vi "Contour Line_Find Candidate Edges.vi"(11 "edge":T2) -> (3 "Candidate Edges":T1(array[cluster]))   [LabVIEW 2020, in "NI_AAL_Geometry.lvlib"]
uses:
  <vilib>/Analysis/NI_AAL_Geometry.lvlib
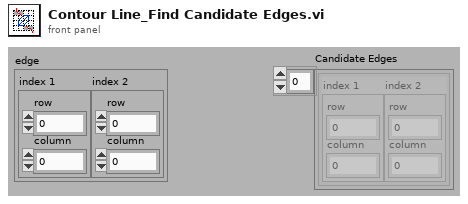
[diagram p1: front panel]
types:
  T1 = cluster{"index 1":cluster{"row":i32, "column":i32}, "index 2":cluster{"row":i32, "column":i32}}[]
  T2 = cluster{"index 1":cluster{"row":i32, "column":i32}, "index 2":cluster{"row":i32, "column":i32}}
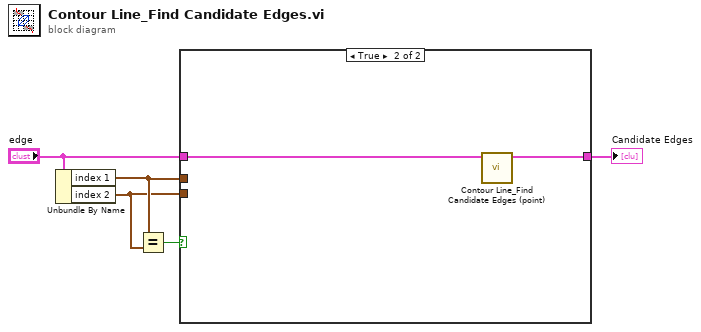
[diagram p0: block diagram]
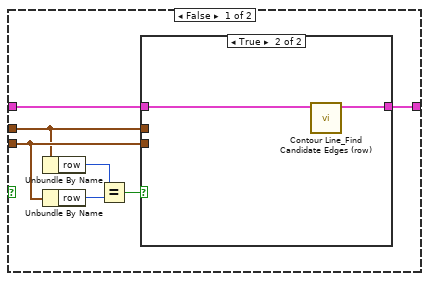
[diagram p2: hidden frame]
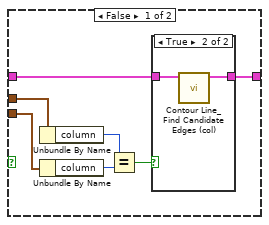
[diagram p3: hidden frame]
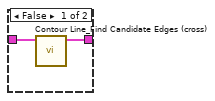
[diagram p4: hidden frame]
diagram:
  n1 = Unbundle By Name("edge") -> ("index 1"=w4:cluster{"row":i32, "column":i32}, "index 2"=w3:cluster{"row":i32, "column":i32})
  n2 = Equal?(x=w4, y=w3) -> (x = y?=w2:bool)
  n3 = case shown="True" w2 {
    tunnel: "edge" -> [w7 w27]
    tunnel: w4 -> [w8 _]
    tunnel: w3 -> [w9 _]
    tunnel: [w6 w26] -> w1
    frame False {
      n4 = Unbundle By Name(w8) -> ("row"=w11:i32)
      n5 = Unbundle By Name(w9) -> ("row"=w12:i32)
      n6 = Equal?(x=w11, y=w12) -> (x = y?=w10:bool)
      n7 = case shown="True" w10 {
        tunnel: w9 -> [w16 _]
        tunnel: w8 -> [w17 _]
        tunnel: w7 -> [w14 w25]
        tunnel: [w13 w24] -> w6
        frame False {
          n8 = Unbundle By Name(w17) -> ("column"=w19:i32)
          n9 = Unbundle By Name(w16) -> ("column"=w18:i32)
          n10 = Equal?(x=w19, y=w18) -> (x = y?=w15:bool)
          n11 = case shown="True" w15 {
            tunnel: w14 -> [w21 w23]
            tunnel: [w20 w22] -> w13
            frame False {
              n12 = call <vilib>:"Contour Line_Find Candidate Edges (cross).vi"("edge"=w21) -> ("Candidate Edges"=w20:T1)  [unwired: 10 out]
            }
            frame True {
              n13 = call <vilib>:"Contour Line_Find Candidate Edges (col).vi"("edge"=w23) -> ("Candidate Edges"=w22:T1)  [unwired: 10 out]
            }
          }
        }
        frame True {
          n14 = call <vilib>:"Contour Line_Find Candidate Edges (row).vi"("edge"=w25) -> ("Candidate Edges"=w24:T1)  [unwired: 10 out]
        }
      }
    }
    frame True {
      n15 = call <vilib>:"Contour Line_Find Candidate Edges (point).vi"("edge"=w27) -> ("Candidate Edges"=w26:T1)  [unwired: 10 out]
    }
  }
  "Candidate Edges" <- w1
